vi "VoltageContinuousOutput_0309_2014ver.vi"() -> ()   [LabVIEW 2014]
doc: "This example demonstrates how to continuously generate an analog output waveform by providing new data to the output buffer as the task is running.\n\nThis example is useful if you want to generate a non-repeating waveform, make updates on-the-fly, or generate a frequency that is not an even divide-down of your sample clock. In this example, the default frequency value is 17 to demonstrate that non-regenerative output can be used to create a signal with a frequency that is not an even divide-down of your sample clock."
uses:
  <resource>/objmgr/daqmx.rc
  <vilib>/measure/NI_MABase.lvlib
  <vilib>/DAQmx/configure/timing.llb/DAQmx Timing (Sample Clock).vi
  <vilib>/DAQmx/create/channels.llb/DAQmx Create Channel (AO-Voltage-Basic).vi
  <vilib>/Utility/error.llb/DialogType.ctl
  <vilib>/DAQmx/configure/trigger.llb/DAQmx Start Trigger (Digital Edge).vi
  <vilib>/DAQmx/configure/trigger.llb/DAQmx Start Trigger (Analog Edge).vi
  <vilib>/DAQmx/configure/trigger.llb/DAQmx Start Trigger (Time).vi
  <vilib>/DAQmx/write.llb/DAQmx Write (Analog 1D Wfm NChan NSamp).vi
panel:
  in  "Trigger Type":T1(tab)
  in  "Digital Start Trigger Edge":i32(ring)=10280 caption="Edge" items=["Rising"=10280, "Falling"=10171]
  in  "Digital Start Trigger Source":tag="/Dev1/PFI0" caption="Source"
  in  "Digital Pause Trigger Pause When":i32(ring)=10192 caption="Pause When" items=["High"=10192, "Low"=10214]
  in  "Digital Pause Trigger Source":tag="/Dev1/PFI0" caption="Source"
  in  "Analog Start Trigger Level":dbl caption="Level" format="%0.2f"
  in  "Analog Start Trigger Hysteresis":dbl caption="Hysteresis" format="%.2f"
  in  "Analog Start Trigger Slope":i32(ring)=10280 caption="Slope" items=["Rising"=10280, "Falling"=10171]
  in  "Analog Start Trigger Source":string="APFI0" caption="Source"
  in  "Analog Pause Trigger Source":string="APFI0" caption="Source"
  in  "Analog Pause Trigger Pause When":i32(ring)=10093 caption="Pause When" items=["Above Level"=10093, "Below Level"=10107]
  in  "Analog Pause Trigger Level":dbl caption="Level" format="%.2f"
  in  "When":timestamp
  in  "Select Time\nManually":bool
  in  "Output Array":T2(array[cluster])=[{"Waveform Type"=0, "Amplitude"=1.0, "Frequency"=17.0, "Phase"=17.0}] {"Phase" format="%0.2p"; "Frequency" format="%0.2p"; "Amplitude" format="%0.2p"; "Waveform Type" items=["Sine Wave", "Triangle Wave", "Square Wave", "Sawtooth Wave"]}
  in  "Number of Samples":i32=1000
  in  "Stop":bool
  out "Waveform Graph":waveform(dbl)[](graph)=[{"t0"=timestamp(0 s since 1904-01-01), "dt"=0.001, "Y"=[]}]
  in  "Sample Rate":dbl=1000.0
  in  "Sample Clock Source":tag="OnboardClock"
  in  "Max Voltage":dbl=5.0
  in  "Min Voltage":dbl=-5.0
  in  "Physical Channel(s)":tag="Dev1/ao0"
  out "Actual Sample Rate":dbl=1000.0 format="%0.2f"
  # "Channel Settings"
  # "Output"
  # "Timing and Buffer Settings"
  # "Waveform Settings"
  # "Trigger Settings"
  # "The number of elements in the waveform array\nmust equal the number of channels in the task."
  # "To enable triggers, select a tab above, and configure the settings.\n\nNot all hardware supports all trigger types. Refer to your device documentation for more information."
  # "This trigger type is not supported in output tasks. \n\nRefer to your device documentation for more information on which triggers are supported."
  # "This trigger type is not supported in output tasks. \n\nRefer to your device documentation for more information on which triggers are supported."
  # "If time is not manually set, task will begin after 10 seconds"
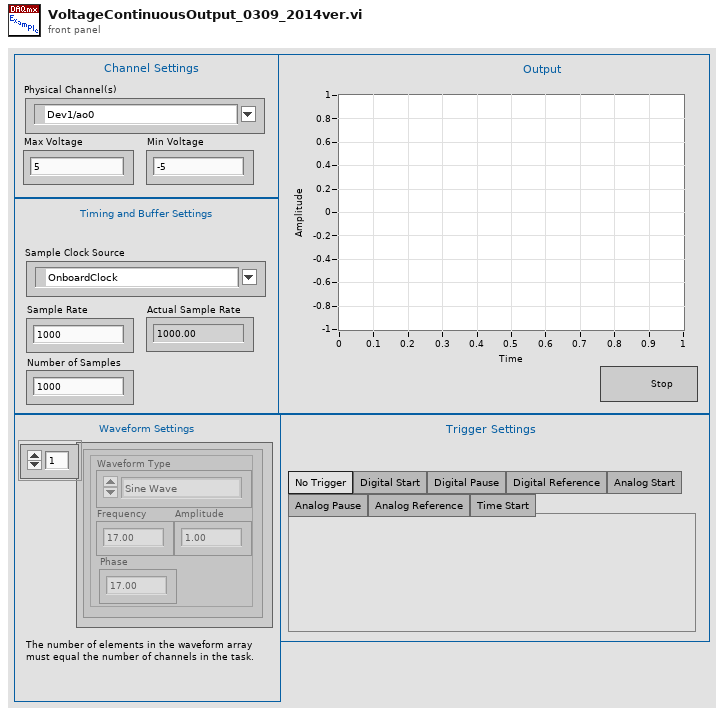
[diagram p1: front panel]
types:
  T1 = enum32{"No Trigger", "Digital Start", "Digital Pause", "Digital Reference", "Analog Start", "Analog Pause", "Analog Reference", "Time Start"}
  T2 = cluster{"Waveform Type":u16, "Amplitude":dbl, "Frequency":dbl, "Phase":dbl}[]
  T3 = typedef "DialogType.ctl" = u16
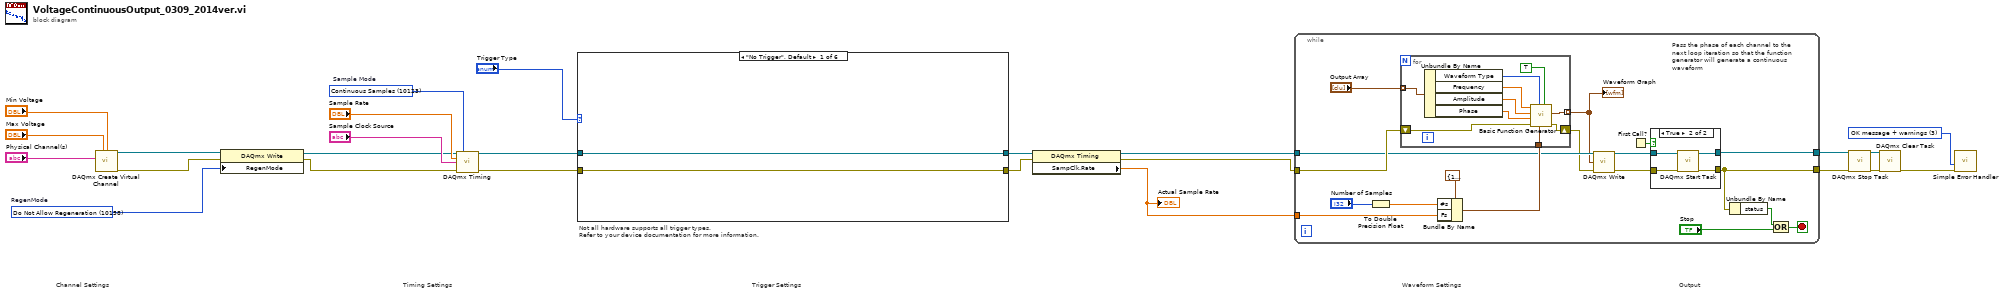
[diagram p0: block diagram]
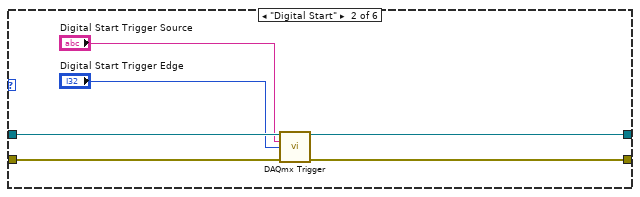
[diagram p2: hidden frame]
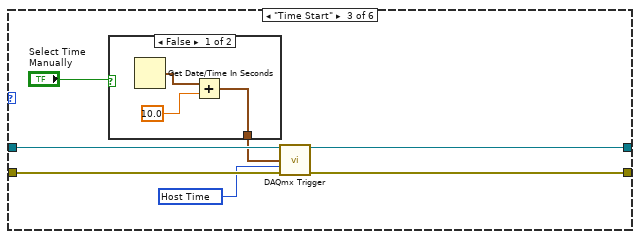
[diagram p3: hidden frame]
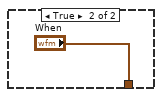
[diagram p4: hidden frame]
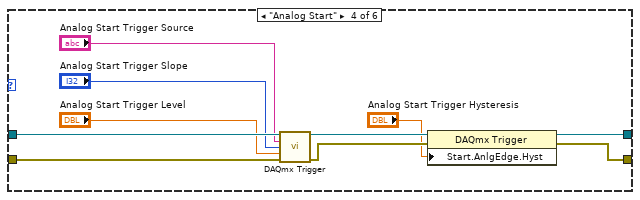
[diagram p5: hidden frame]
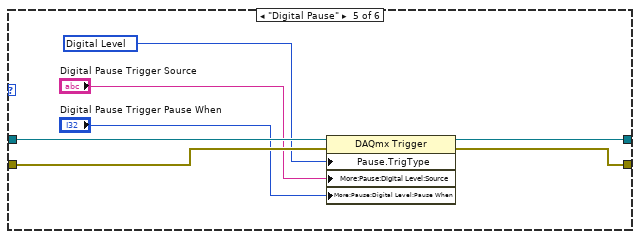
[diagram p6: hidden frame]
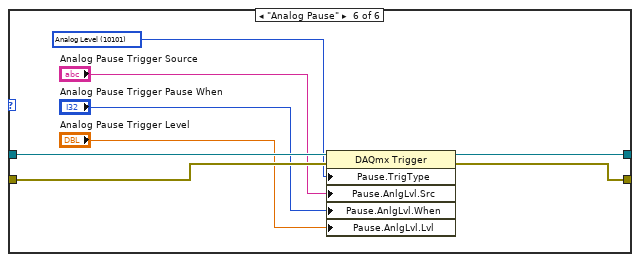
[diagram p7: hidden frame]
diagram:
  w8 = T3 3 items=["no dialog", "OK message", "continue or stop message", "OK message + warnings", "continue/stop + warnings"] ("type of dialog (OK msg:1)")
  w15 = 10158 items=["Allow Regeneration"=10097, "Do Not Allow Regeneration"=10158]  # RegenMode
  w25 = 10123 items=["Finite Samples"=10178, "Continuous Samples"=10123, "Hardware Timed Single Point"=12522]  # Sample Mode
  # "Trigger Settings"
  # "Not all hardware supports all trigger types.\nRefer to your device documentation for more information."
  # "Output"
  # "Waveform Settings"
  # "Timing Settings"
  # "Channel Settings"
  n1 = call-poly <vilib>:"DAQmx Create Virtual Channel.vi"("maximum value"="Max Voltage", "minimum value"="Min Voltage", "physical channels"="Physical Channel(s)") -> ("task out"=w17:refnum<k21>, "error out"=w16:errorcluster)  [unwired: 11 in]
  n2 = property class="DAQmx Write"(reference=w17, error in=w16, "RegenMode"=w15) -> (reference out=w13:refnum<k21>, error out=w14:errorcluster)
  n3 = call-poly <vilib>:"DAQmx Timing.vi"("task/channels in"=w13, "sample mode"=w25, "rate"="Sample Rate", "source"="Sample Clock Source", "error in"=w14) -> ("task out"=w5:refnum<k21>, "error out"=w6:errorcluster)  [unwired: 9 in]
  n4 = case shown="\"No Trigger\", Default" "Trigger Type" {
    tunnel: w5 -> [w27 w33 w40 w54 w61 w69]
    tunnel: w6 -> [w26 w32 w39 w53 w58 w66]
    tunnel: [w27 w31 w38 w51 w60 w68] -> w4
    tunnel: [w26 w30 w37 w50 w59 w67] -> w3
    frame "No Trigger", Default {
    }
    frame "Digital Start" {
      n5 = call-poly <vilib>:"DAQmx Trigger.vi"("task/channels in"=w33, "source"="Digital Start Trigger Source", "edge"="Digital Start Trigger Edge", "error in"=w32) -> ("task out"=w31:refnum<k21>, "error out"=w30:errorcluster)  [unwired: 10 in]
    }
    frame "Time Start" {
      w34 = 16126 items=["Host Time"=16126, "I/O Device Time"=16127] ("timescale")
      n6 = case shown="False" "Select Time\nManually" {
        tunnel: [w42 "When"] -> w35
        frame False {
          n7 = Get Date/Time In Seconds() -> (seconds since 1Jan1904=w43:timestamp)
          n8 = Add(x=w43, y=10.0) -> (x+y=w42:timestamp)
        }
        frame True {
        }
      }
      n9 = call-poly <vilib>:"DAQmx Trigger.vi"("task/channels in"=w40, "when"=w35, "timescale"=w34, "error in"=w39) -> ("task out"=w38:refnum<k21>, "error out"=w37:errorcluster)  [unwired: 10 in]
    }
    frame "Analog Start" {
      n10 = call-poly <vilib>:"DAQmx Trigger.vi"("task/channels in"=w54, "source"="Analog Start Trigger Source", "slope"="Analog Start Trigger Slope", "level"="Analog Start Trigger Level", "error in"=w53) -> ("task out"=w49:refnum<k21>, "error out"=w48:errorcluster)  [unwired: 9 in]
      n11 = property class="DAQmx Trigger"(reference=w49, error in=w48, "Start.AnlgEdge.Hyst"="Analog Start Trigger Hysteresis") -> (reference out=w51:refnum<k21>, error out=w50:errorcluster)
    }
    frame "Digital Pause" {
      w57 = 10152 items=["Analog Level"=10101, "Analog Window"=10103, "Digital Level"=10152, "Digital Pattern"=10398, "None"=10230] ("Pause.TrigType")
      n12 = property class="DAQmx Trigger"(reference=w61, error in=w58, "Pause.TrigType"=w57, "More:Pause:Digital Level:Source"="Digital Pause Trigger Source", "More:Pause:Digital Level:Pause When"="Digital Pause Trigger Pause When") -> (reference out=w60:refnum<k21>, error out=w59:errorcluster)
    }
    frame "Analog Pause" {
      w65 = 10101 items=["Analog Level"=10101, "Analog Window"=10103, "Digital Level"=10152, "Digital Pattern"=10398, "None"=10230] ("Pause.TrigType")
      n13 = property class="DAQmx Trigger"(reference=w69, error in=w66, "Pause.TrigType"=w65, "Pause.AnlgLvl.Src"="Analog Pause Trigger Source", "Pause.AnlgLvl.When"="Analog Pause Trigger Pause When", "Pause.AnlgLvl.Lvl"="Analog Pause Trigger Level") -> (reference out=w68:refnum<k21>, error out=w67:errorcluster)
    }
  }
  n14 = property class="DAQmx Timing"(reference=w4, error in=w3) -> (reference out=w2:refnum<k21>, error out=w1:errorcluster, "SampClk.Rate"=w18:dbl)
  "Actual Sample Rate" <- w18
  n15 = while {
    tunnel: w1 -> [w87]
    tunnel: w18 -> [w85]
    tunnel: w2 -> [w83]
    tunnel: [w75] -> w10
    tunnel: [w74] -> w9
    stop <- w72 stop-if-true
    # "Pass the phase of each channel to the next loop iteration so that the function generator will generate a continuous waveform"
    n16 = To Double Precision Float(number="Number of Samples") -> (double precision float=w78:dbl)
    n17 = Bundle By Name(cluster=cluster{"Fs":dbl, "#s":dbl} {"Fs"=1000.0, "#s"=1000.0} ("sampling info"), "#s"=w78, "Fs"=w85) -> (w84:cluster{"Fs":dbl, "#s":dbl})
    n18 = for {
      tunnel: w84 -> [w102]
      tunnel: "Output Array" -> [w100] mode=indexing
      tunnel: [w96] -> w70 mode=indexing
      shift-right: [w101] -> w80
      shift-left: w87 -> [w103]
      n19 = Unbundle By Name(w100) -> ("Waveform Type"=w99:u16, "Frequency"=w98:dbl, "Amplitude"=w97:dbl, "Phase"=w94:dbl)
      n20 = call <vilib>:"Basic Function Generator.vi"("reset signal"=TRUE, "sampling info"=w102, "signal type"=w99, "error in (no error)"=w103, "phase"=w94, "amplitude"=w97, "frequency"=w98) -> ("error out"=w101:errorcluster, "signal out"=w96:waveform(dbl))  [unwired: 2 in, 1 out]
    }
    "Waveform Graph" <- w70
    n21 = call-poly <vilib>:"DAQmx Write.vi"("task/channels in"=w83, "data"=w70, "error in"=w80) -> ("task out"=w82:refnum<k21>, "error out"=w81:errorcluster)  [unwired: 10 in, 1 out]
    n22 = First Call?() -> (First Call?: T/F=w76:bool)
    n23 = case shown="True" w76 {
      tunnel: w82 -> [w88 w93]
      tunnel: w81 -> [w89 w92]
      tunnel: [w88 w91] -> w75
      tunnel: [w89 w90] -> w74
      frame False {
      }
      frame True {
        n24 = call <vilib>:"DAQmx Start Task.vi"("task/channels in"=w93, "error in"=w92) -> ("task out"=w91:refnum<k21>, "error out"=w90:errorcluster)  [unwired: 12 in]
      }
    }
    n25 = Unbundle By Name(w74) -> ("status"=w71:bool)
    n26 = Or(x=w71, y="Stop") -> (x .or. y?=w72:bool)
  }
  n27 = call <vilib>:"DAQmx Stop Task.vi"("task/channels in"=w10, "error in"=w9) -> ("task out"=w12:refnum<k21>, "error out"=w11:errorcluster)  [unwired: 12 in]
  n28 = call <vilib>:"DAQmx Clear Task.vi"("task in"=w12, "error in"=w11) -> ("error out"=w24:errorcluster)  [unwired: 13 in]
  n29 = call <vilib>:"Simple Error Handler.vi"("type of dialog (OK msg:1)"=w8, "error in (no error)"=w24) -> ()  [unwired: 3 in, 5 out]
